vi "Resave Setup file PM Only.vi"() -> (0 "PM index":i32[](array[numeric]), 1 "Setup filename":string="Pressure_Multiplexer_Remote_Setup.xls")   [LabVIEW 2022 SP3]
uses:
  File/Setup_Filetype.ctl
  Globals/Meas_global.vi
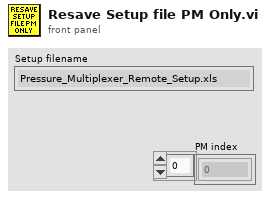
[diagram p1: front panel]
types:
  T1 = typedef "Setup_Filetype.ctl" = enum16{"Measurement Setups", "Calibration Setups", "General", "Results File Plotter Setups", "Speed Calib Tweaks"}
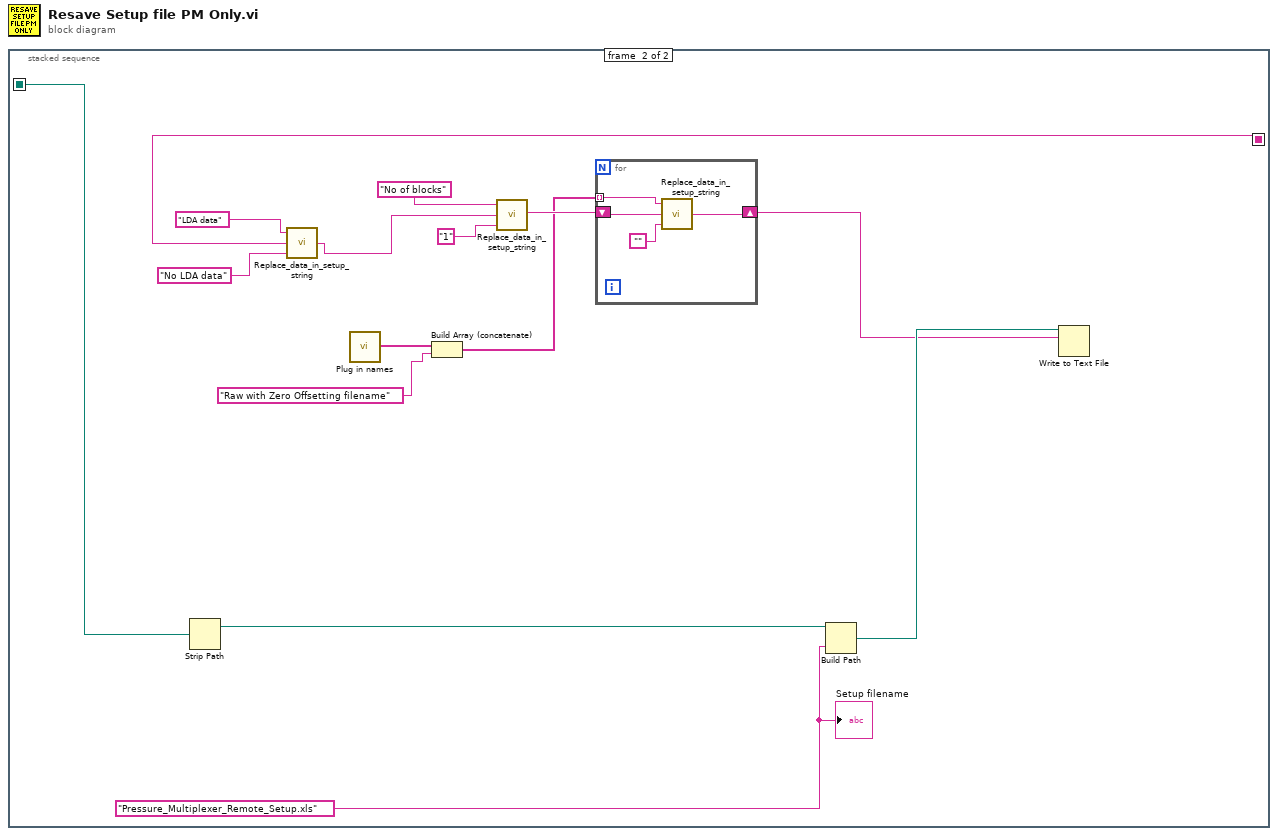
[diagram p0: block diagram]
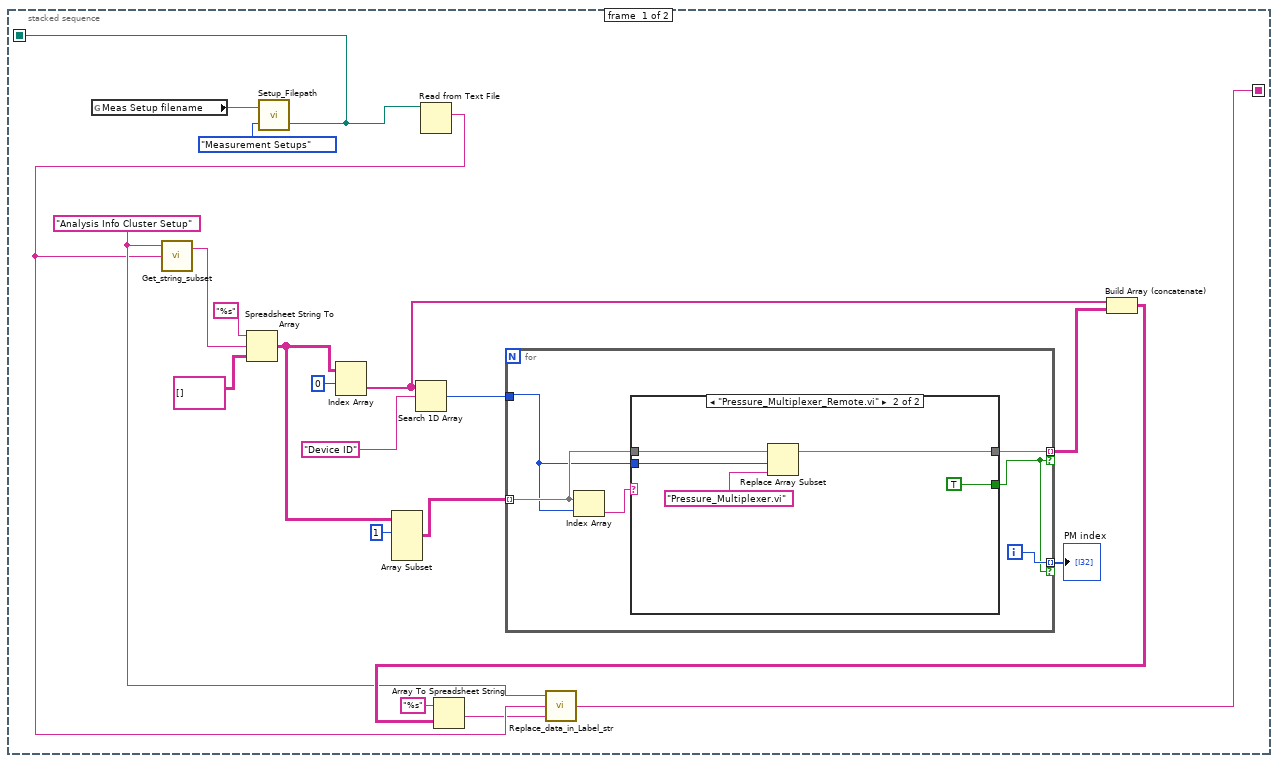
[diagram p2: hidden frame]
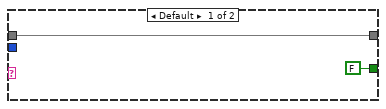
[diagram p3: hidden frame]
diagram:
  n1 = stacked-sequence {
    seq-local: [w3 _] -> [_ w49]
    seq-local: [w2 _] -> [_ w46]
    frame #0 {
      w6 = "Analysis Info Cluster Setup"
      n2 = global read "Meas_global.vi" "Meas Setup filename"() -> (w20:string)
      n3 = call "Setup_Filepath.vi"("Setup File Type"=Setup_Filetype."Measurement Setups", "Filename in"=w20) -> ("Filename Out"=w2:path)  [unwired: 1 out]
      n4 = Read from Text File(file (use dialog)=w2) -> (text=w5:string)  [unwired: 3 in, 3 out]
      n5 = call "Get_string_subset.vi"("String to split"=w5, "File Label"=w6) -> ("Output string"=w17:string)  [unwired: 2 in, 1 out]
      n6 = Spreadsheet String To Array(format string="%s", spreadsheet string=w17, array type (2D Dbl)=string[][] []) -> (array=w14:string[][])  [unwired: 1 in]
      n7 = Index Array(array=w14, index (row)=0) -> (element=w9:string[])  [unwired: 1 in]
      n8 = Array Subset(array=w14, index (row)=1 ("index")) -> (w11:string[][])  [unwired: 3 in]
      n9 = Search 1D Array(1D array=w9, element="Device ID") -> (index of element=w12:i32)  [unwired: 1 out]
      n10 = for {
        tunnel: w12 -> [w25]
        tunnel: w11 -> [w26] mode=indexing
        tunnel: [w24] -> w10 mode=indexing if=w22
        tunnel: [w23] -> w1 mode=indexing if=w22
        i -> [w23]
        n11 = Index Array(array=w26, index=w25) -> (element=w27:string)
        n12 = case shown="\"Pressure_Multiplexer_Remote.vi\"" w27 {
          tunnel: w26 -> [w28 w34]
          tunnel: w25 -> [_ w33]
          tunnel: [w28 w31] -> w24
          tunnel: [FALSE TRUE] -> w22
          frame Default {
          }
          frame "Pressure_Multiplexer_Remote.vi" {
            n13 = Replace Array Subset(array=w34, new element="Pressure_Multiplexer.vi", index=w33) -> (w31:string[])
          }
        }
      }
      "PM index" <- w1
      n14 = Build Array (concatenate)(w9, w10) -> (w7:string[][])
      n15 = Array To Spreadsheet String(array=w7, 3:"%s" ("format string")) -> (spreadsheet string=w4:string)  [unwired: 1 in]
      n16 = call "Replace_data_in_Label_str.vi"("New data string"=w4, "Input string"=w5, "Variable name"=w6) -> ("Appended string"=w3:string)
    }
    frame #1 {
      w44 = "Pressure_Multiplexer_Remote_Setup.xls"
      n17 = Strip Path(path=w46) -> (stripped path=w45:path)  [unwired: 1 out]
      n18 = call "Replace_data_in_setup_string.vi"("New data string"="No LDA data", "Input string"=w49, "Variable name"="LDA data" ("Label for characters")) -> ("Appended string"=w42:string)
      n19 = call "Plug in names.vi"() -> ("Array"=w37:string[])  [unwired: 1 in]
      n20 = Build Array (concatenate)(w37, "Raw with Zero Offsetting filename" ("Label for characters")) -> (w36:string[])
      n21 = call "Replace_data_in_setup_string.vi"("New data string"="1", "Input string"=w42, "Variable name"="No of blocks") -> ("Appended string"=w39:string)
      n22 = for {
        shift-right: [w51] -> w38
        shift-left: w39 -> [w52]
        tunnel: w36 -> [w50] mode=indexing
        n23 = call "Replace_data_in_setup_string.vi"("New data string"="", "Input string"=w52, "Variable name"=w50) -> ("Appended string"=w51:string)
      }
      n24 = Build Path(base path=w45, name or relative path=w44) -> (appended path=w43:path)
      n25 = Write to Text File(file (use dialog)=w43, text=w38) -> ()  [unwired: 2 in, 3 out]
      "Setup filename" <- w44
    }
  }
